vi "Initialize.vi"(8 "error in (no error)":errorcluster, 9 "Control Properties":T1(array[cluster]), 10 "VI Refnum":refnum<vi>, 11 "CD Parameter Manager in":refnum<class "CD Parameter Manager.lvclass">) -> (0 "error out":errorcluster, 3 "CD Parameter Manager out":refnum<class "CD Parameter Manager.lvclass">)   [LabVIEW 2016, in "CD Parameter Manager API.lvlib" / "CD Parameter Manager.lvclass"]
uses:
  CD Parameter Manager.lvclass
  I32 Parameter Class/I32 Parameter.lvclass
  Boolean Parameter Class/Boolean Parameter.lvclass
  Double Parameter Class/Double Parameter.lvclass
  Parameter Class/Parameter.lvclass
  String Parameter Class/String Parameter.lvclass
  File Path Parameter Class/File Path Parameter.lvclass
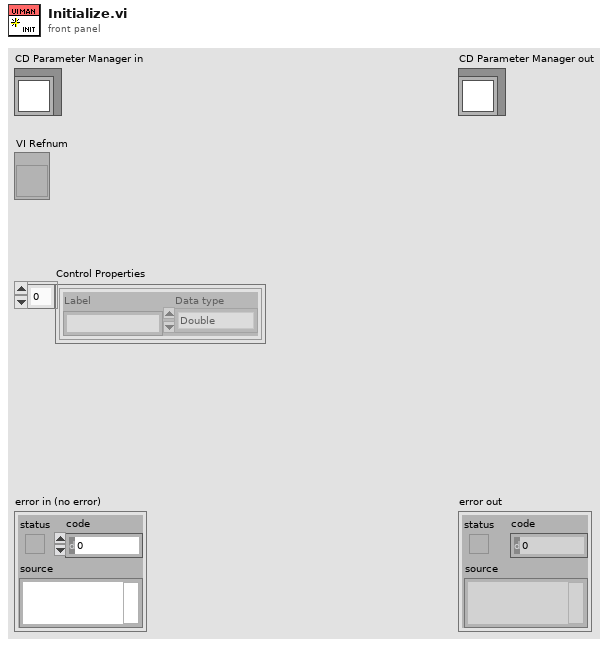
[diagram p1: front panel]
types:
  T1 = cluster{"Label":string, "Data type":enum16{"Double", "I32", "Boolean", "String", "File Path"}}[]
  T2 = enum16{"Double", "I32", "Boolean", "String", "File Path"}
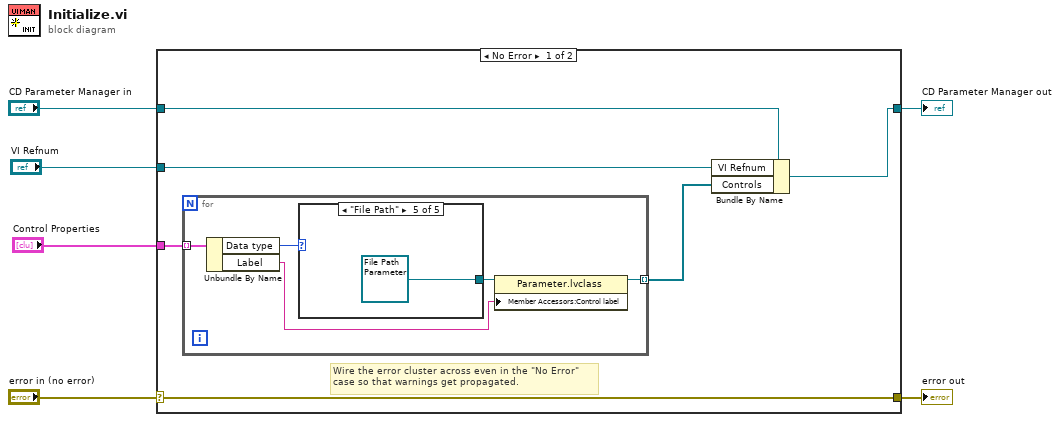
[diagram p0: block diagram]
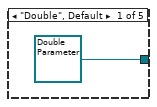
[diagram p2: hidden frame]
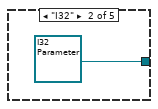
[diagram p3: hidden frame]
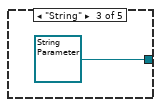
[diagram p4: hidden frame]
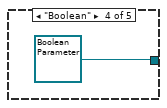
[diagram p5: hidden frame]
diagram:
  n1 = case shown="No Error" "error in (no error)" {
    selector: "error in (no error)" -> [w12 w24]
    tunnel: [w12 w24] -> w5
    tunnel: [w9 w23] -> w3
    tunnel: "CD Parameter Manager in" -> [w11 w23]
    tunnel: "VI Refnum" -> [w10 _]
    tunnel: "Control Properties" -> [w8 _]
    frame No Error {
      # "Wire the error cluster across even in the \"No Error\"\ncase so that warnings get propagated."
      n2 = for {
        tunnel: w8 -> [w17] mode=indexing
        tunnel: [w14] -> w7 mode=indexing
        n3 = Unbundle By Name(w17) -> ("Data type"=w16:T2, "Label"=w13:string)
        n4 = case shown="\"File Path\"" w16 {
          tunnel: [refnum<class "Double Parameter.lvclass"> refnum ("CD Parameter Manager API.lvlib:Double Parameter.lvclass") refnum<class "I32 Parameter.lvclass"> refnum ("CD Parameter Manager API.lvlib:I32 Parameter.lvclass") refnum<class "String Parameter.lvclass"> refnum ("CD Parameter Manager API.lvlib:String Parameter.lvclass") refnum<class "Boolean Parameter.lvclass"> refnum ("CD Parameter Manager API.lvlib:Boolean Parameter.lvclass") refnum<class "File Path Parameter.lvclass"> refnum ("CD Parameter Manager API.lvlib:File Path Parameter.lvclass")] -> w15
          frame "Double", Default {
          }
          frame "I32" {
          }
          frame "String" {
          }
          frame "Boolean" {
          }
          frame "File Path" {
          }
        }
        n5 = property class="Parameter.lvclass"(reference=w15, "Member Accessors:Control label"=w13) -> (reference out=w14:refnum<class "Parameter.lvclass">)  [unwired: 1 in, 1 out]
      }
      n6 = Bundle By Name(cluster=w11, "VI Refnum"=w10, "Controls"=w7) -> (w9:refnum<class "CD Parameter Manager.lvclass">)
    }
    frame Error {
    }
  }
  "error out" <- w5
  "CD Parameter Manager out" <- w3
